vi "Measurement UI.vi"() -> ()   [LabVIEW 2023, in "FPT NoiseFigure UI.lvlib"]
uses:
  FPT NoiseFigure UI.lvlib
  <vilib>/Utility/file.llb/Read Delimited Spreadsheet (DBL).vi
panel:
  in  "Measurement Graph":enum32{"DUT NF", "Separated", "Hidden Controls"}(tab)
  out "Combined Graph":T1(graph)
  out "Graph 2":T1(graph)
  out "Graph 1":T1(graph)
  in  "Power sequencing file validity check":bool=TRUE
  in  "ENS SMU Name":string="5842_0"
  out "DUT NF (mean)":dbl format="%.2g"
  in  "Noise Source Loss S2P File Path":string
  in  "Calibration Loss S2P File Path":string
  in  "DUT Output Loss S2P File Path":string
  in  "DUT Input Loss S2P File Path":string
  out "Analyzer NF vs Freq":dbl[][](array[numeric]) format="%.2g"
  out "DUT NF vs Freq":dbl[][](array[numeric]) format="%.2g"
  in  "Power sequencing file path":string
  in  "RFmx name":string="5842_0"
  in  "RFmx attenuation mode":T2(ring)=enum."Constant Attenuation"
  in  "RFmx s2p file path":string
  out "All Graph Refs":refnum<vi>[](array[refnum])
  in  "ENR Freq (Hz)":dbl[](array[numeric])=[6500000000.0] caption="ENR Freq" format="%.3p Hz"
  in  "ENR (dB)":dbl[](array[numeric])=[15.0] caption="ENR" format="%.2g dB"
  out "Analyzer NF(s)":string[](array[string])
  out "DUT NF(s)":string[](array[string])
  out "Frequencies":string[](array[string])
  out "DUT NF (Mean)":string[](array[string])
  in  "Noise Source Type":i32(ring)=1 items=["External Noise Source", "RF Signal Generator"]
  in  "Switch Name":string
  out "MeasTable 1":string[][](table)
  out "MeasTable 2":string[][](table)
  in  "Action":u32(ring) items=["Measure", "Calibrate"]
  in  "Mode of operation":T3(ring) caption="Configuration"
  in  "Tab Control":T4(tab)
  in  "Power sequencing file path_update":path caption="Power Sequencing File Path"
  in  "RFmx port":string(combo)="port2" caption="RFmx Port"
  in  "RFmx attenuation mode_tab":T2(tab)=enum."s2p File" caption="RFmx Attenuation Mode"
  in  "RFmx external attenuation (dB)":dbl=0.8 caption="External Attenuation" format="%#fdB"
  in  "RFmx s2p file path_update":path caption="S2P File Path"
  in  "RFmx s-parameters orientation":enum32{"Port1 Towards DUT", "Port2 Towards DUT"}(ring) caption="Orientation"
  in  "RFmx name_update":refnum<k15> caption="RFmx Name"
  in  "DUT Output_Orientation":enum32{"Port1 Towards DUT", "Port2 Towards DUT"}(ring) caption="Orientation"
  in  "DUT Input_Orientation":enum32{"Port1 Towards DUT", "Port2 Towards DUT"}(ring) caption="Orientation"
  in  "DUT Output_Compensation Enabled":bool caption="Enabled"
  in  "DUT Input_Compensation Enabled":bool caption="Enabled"
  in  "DUT Input_Temperation (K)":dbl=297.0 caption="Temperature" format="%#fK"
  in  "DUT Output_Temperation (K)":dbl=297.0 caption="Temperature" format="%#fK"
  in  "DUT Input_Loss S2P":path=path "C:/Users/ies-pg-8881/Desktop/KB/CMT/PS_ATT6dB_26.5GHz.csv" caption="DUT Input Loss S2P"
  in  "DUT Output_Loss S2P":path=path "C:/Users/ies-pg-8881/Desktop/KB/CMT/PS_ATT6dB_26.5GHz.csv" caption="DUT Output Loss S2P"
  in  "Noise Source_Orientation":enum32{"Port1 Towards DUT", "Port2 Towards DUT"}(ring) caption="Orientation"
  in  "Calibration_Orientation":enum32{"Port1 Towards DUT", "Port2 Towards DUT"}(ring) caption="Orientation"
  in  "Noise Source_Compensation Enabled":bool caption="Enabled"
  in  "Calibration_Temperation (K)":dbl=297.0 caption="Temperature" format="%#fK"
  in  "Noise Source_Temperation (K)":dbl=297.0 caption="Temperature" format="%#fK"
  in  "Calibration_Compensation Enabled":bool caption="Enabled"
  in  "Calibration_Loss S2P":path=path "C:/Users/ies-pg-8881/Desktop/KB/CMT/PS_ATT6dB_26.5GHz.csv" caption="Calibration Loss S2P"
  in  "Noise Source_Loss S2P":path=path "C:/Users/ies-pg-8881/Desktop/KB/CMT/PS_ATT6dB_26.5GHz.csv" caption="Noise Source Loss S2P"
  in  "Noise Source Type_Tab":T5(tab)=enum."RF Signal Generator" caption="Noise Source Type"
  in  "ENS SMU Channel":string
  in  "ENS SMU name_update":refnum<k15> caption="ENS SMU Name"
  in  "Switch Connection":string
  in  "Switch Name_update":refnum<k15> caption="Switch Name"
  in  "Noise Source RFSG Port":string(combo)="port1" caption="RFSG Port"
  in  "ENR_File Path":path caption="ENR File Path"
  in  "ENR_Values":cluster{"Frequency":dbl, "Value":dbl}[](array[cluster])=[{"Frequency"=6500000000.0, "Value"=15.0}] {"Value" format="%#fdB"; "Frequency" format="%#pHz"}
  in  "Noise Source Off Temperature (K)":dbl=297.0 caption="Off Temp" format="%#fK"
  in  "Noise Source Cold Temperature (K)":dbl=302.8 caption="Cold Temp" format="%#fK"
  in  "Averaging Enabled":bool
  in  "NF Cal Setup ID":string="SNS_PS_6dB_ENR15_26.5GHz_VI" caption="Calibration Setup ID"
  in  "Preamp Enabled":i32(ring)=3 caption="Preamp" items=["Disabled"=0, "Enabled"=1, "Automatic"=3]
  in  "Reference Level (dBm)":dbl caption="Reference Level" format="%#fdBm"
  in  "Reference Level Mode":enum32{"Manual", "Recommend"}(ring)=enum."Recommend"
  in  "DUT Max Noise Figure (dB)":dbl=3.0 caption="DUT Max Noise Figure" format="%#fdB"
  in  "DUT Max Gain (dB)":dbl=17.5 caption="DUT Max Gain" format="%#fdB"
  in  "Measurement Interval (s)":dbl=0.1 caption="Measurement Interval" format="%#ps"
  in  "Measurement Bandwidth (Hz)":dbl=4000000.0 caption="Measurement BW" format="%#pHz"
  in  "Averaging Count":i32=10
  in  "Frequency List Mode":enum32{"Step", "Points", "Frequency List"}(tab) caption="De-embedding"
  in  "Step - Start Frequency":dbl=4000000000.0 caption="Start Frequency" format="%#pHz"
  in  "Step - Stop Frequency":dbl=20000000000.0 caption="Stop Frequency" format="%#pHz"
  in  "Step - Step Size":dbl=1000000000.0 caption="Step Size" format="%#pHz"
  in  "Points - Number of Points":i32=11 caption="Number of Points"
  in  "Points - Stop Frequency":dbl=20000000000.0 caption="Stop Frequency" format="%#pHz"
  in  "Points - Start Frequency":dbl=4000000000.0 caption="Start Frequency" format="%#pHz"
  in  "FreqList - Frequency List":dbl[](array[numeric]) caption="Frequency List" format="%#pHz"
  out "Status":string
  # "DUT Input Compensation"
  # "DUT Output Compensation"
  # "Calibration Compensation"
  # "Noise Source Compensation"
  # "Noise Source"
  # "ENR Frequency"
  # "ENR"
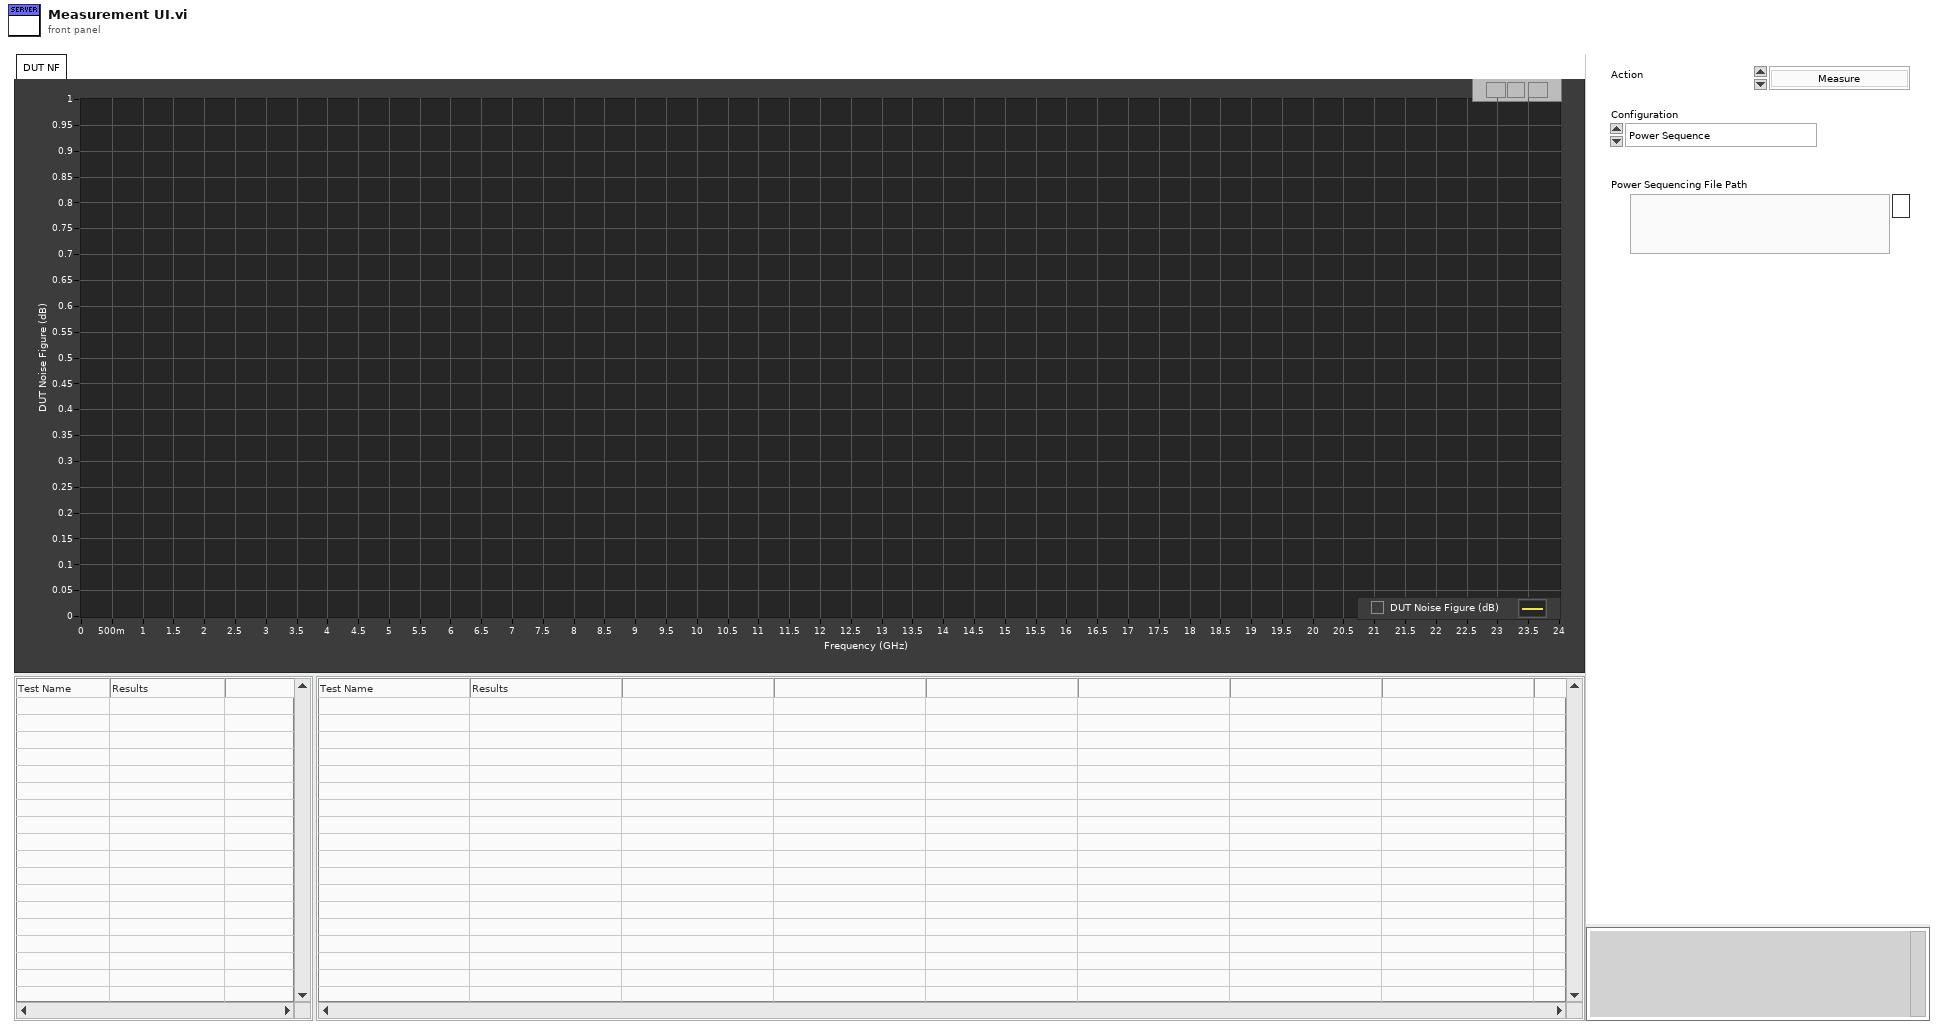
[diagram p1: front panel]
types:
  T1 = cluster{"Load currents":dbl[], "Efficiency":dbl[]}[]
  T2 = enum32{"<None>", "Constant Attenuation", "s2p File"}
  T3 = enum32{"Power Sequence", "HW + De-embedding", "Correction 1", "Correction 2", "Noise Source", "Measurement 1", "Measurement 2"}
  T4 = enum32{"Power Sequence", "De-embedding", "Correction 1", "Correction 2", "Noise Source", "Measurement 1", "Measurement 2"}
  T5 = enum32{"External Noise Source", "RF Signal Generator"}
  T6 = enum16{"<None>", "Constant Attenuation", "s2p File"}
  T7 = enum8{"Enabled", "Disabled", "Disabled and Grayed Out"}
  T8 = cluster{"Shift":bool, "Ctrl":bool, "Alt":bool, "Cmd":bool, "Opt":bool}
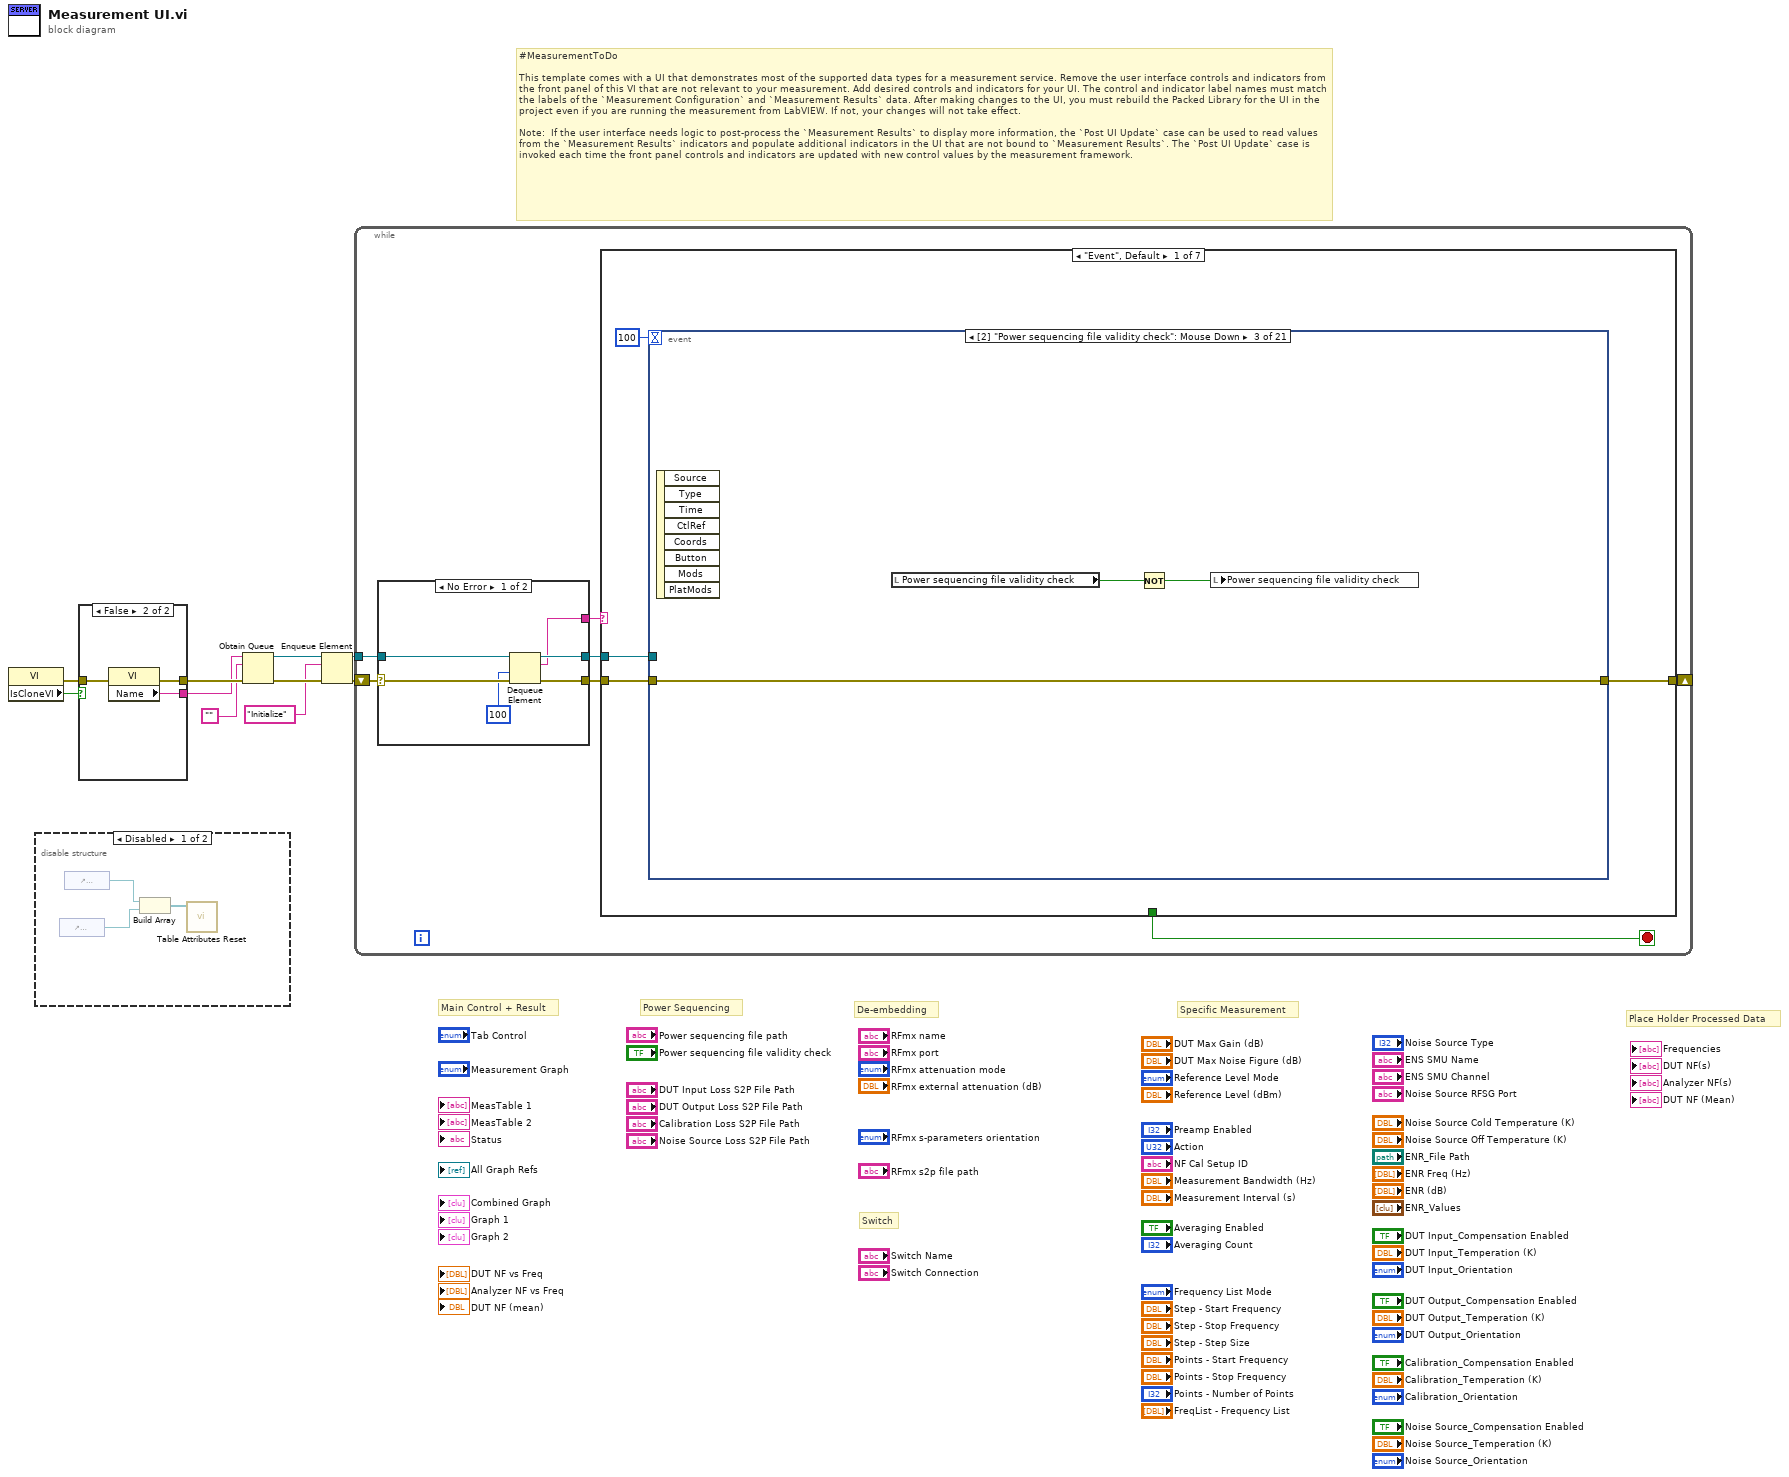
[diagram p0: block diagram]
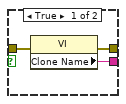
[diagram p3: hidden frame]
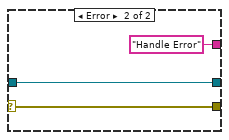
[diagram p4: hidden frame]
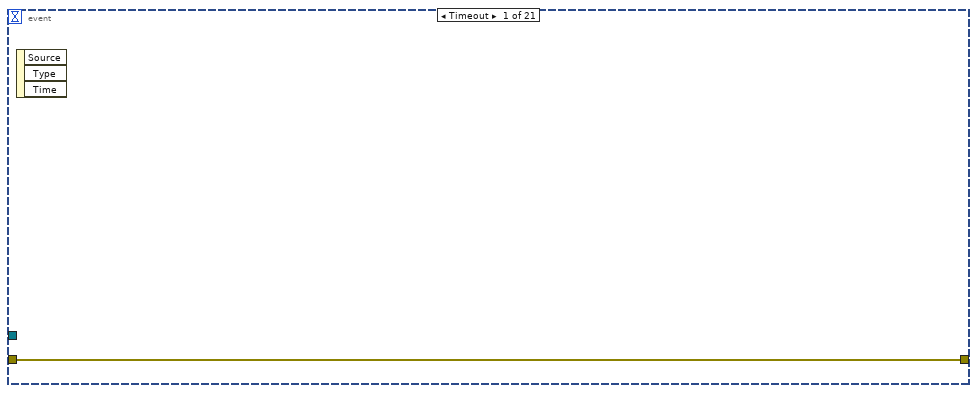
[diagram p5: hidden frame]
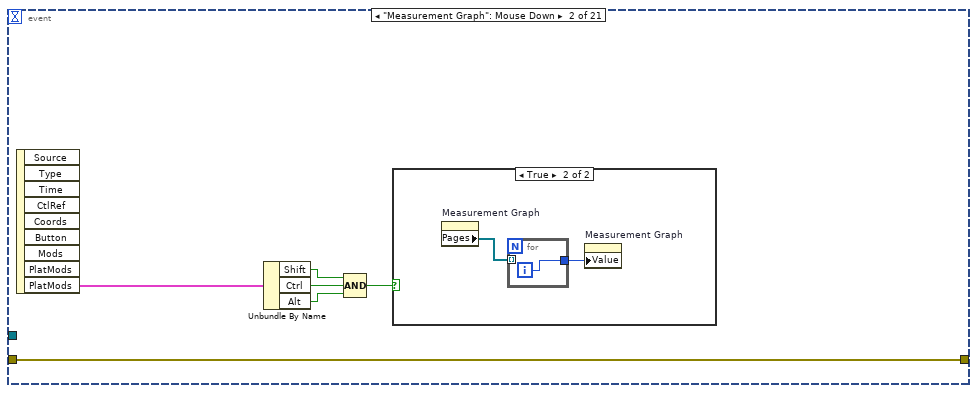
[diagram p6: hidden frame]
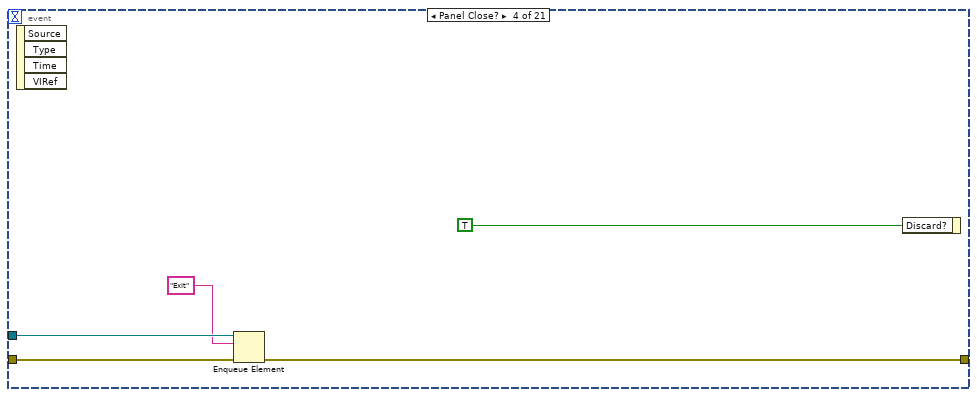
[diagram p8: hidden frame]
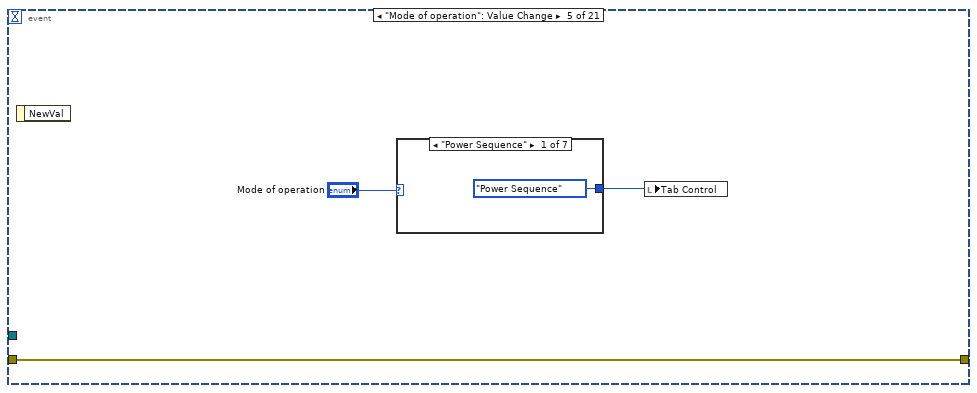
[diagram p9: hidden frame]
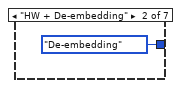
[diagram p10: hidden frame]
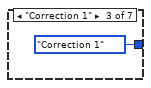
[diagram p11: hidden frame]
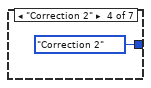
[diagram p12: hidden frame]
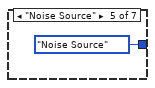
[diagram p13: hidden frame]
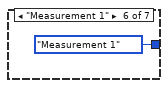
[diagram p14: hidden frame]
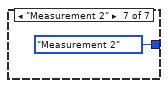
[diagram p15: hidden frame]
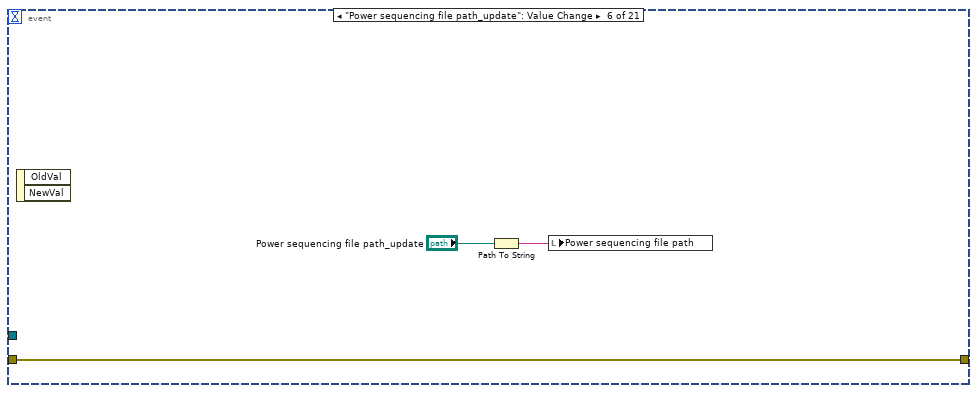
[diagram p16: hidden frame]
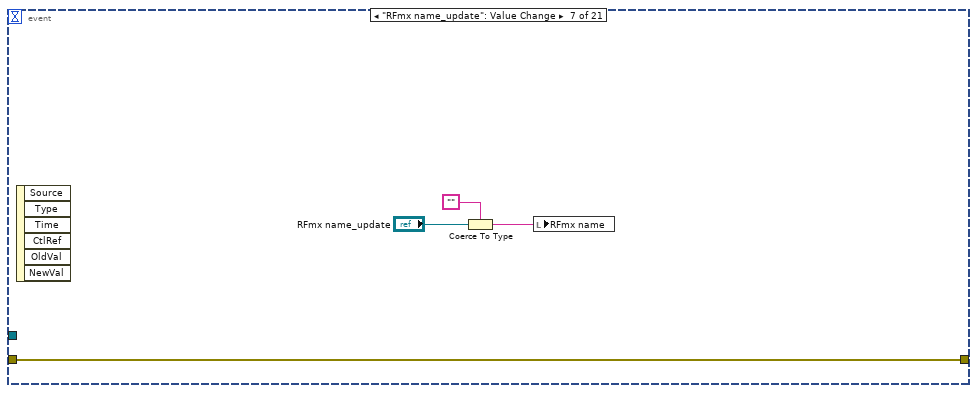
[diagram p17: hidden frame]
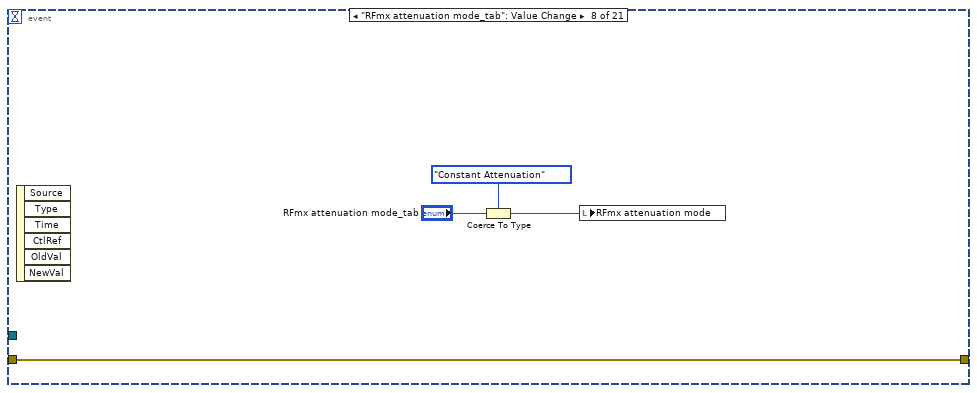
[diagram p18: hidden frame]
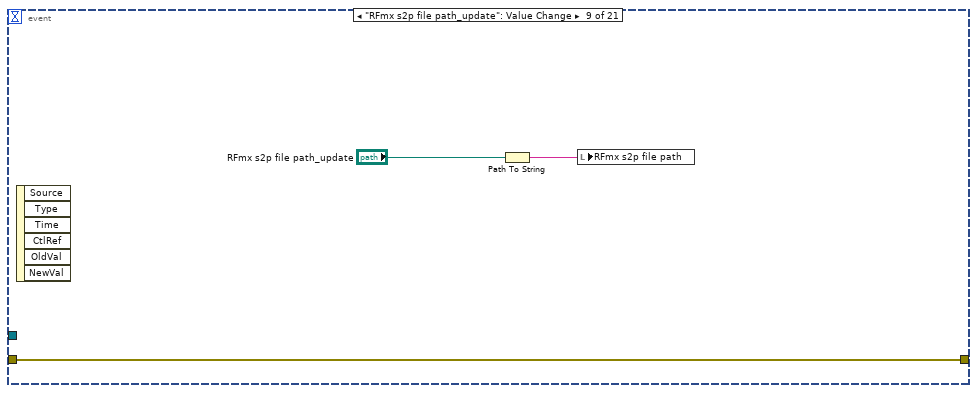
[diagram p19: hidden frame]
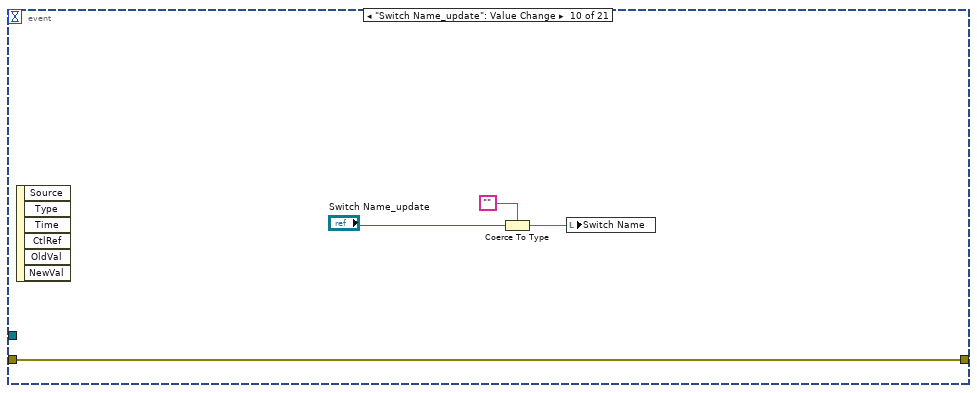
[diagram p20: hidden frame]
diagram:
  # "Switch"
  # "Place Holder Processed Data"
  # "Specific Measurement"
  # "De-embedding"
  # "Power Sequencing"
  # "Main Control + Result"
  # "#MeasurementToDo  \n\nThis template comes with a UI that demonstrates most of the supported data types for a measurement service. Remove the user interface controls and indicators from the front panel of this VI that are not relevant to your measurement. Add desired controls and indicators for your UI. The control and indicator label names must match the labels of the `Measurement Configuration` and `Measurement Results` data. After making changes to the UI, you must rebuild the Packed Library for the UI in the project even if you are running the measurement from LabVIEW. If not, your changes will not take effect.\n\nNote:  If the user interface needs logic to post-process the `Measurement Results` to display more information, the `Post UI Update` case can be used to read values from the `Measurement Results` indicators and populate additional indicators in the UI that are not bound to `Measurement Results`. The `Post UI Update` case is invoked each time the front panel controls and indicators are updated with new control values by the measurement framework."
  n1 = property class="VI"() -> (error out=w1:errorcluster, "IsCloneVI"=w2:bool)  [unwired: 2 in, 1 out]
  n2 = disable-structure shown="Disabled" {
    frame Disabled {
      n3 = control-ref of="MeasTable 2"() -> (w13:refnum<vi>)
      n4 = control-ref of="MeasTable 1"() -> (w12:refnum<vi>)
      n5 = Build Array(w12, w13) -> (w11:refnum<vi>[])
      n6 = call "Table Attributes Reset.vi"("Table Refs"=w11) -> ()  [unwired: 11 in]
    }
    frame Enabled {
    }
  }
  n7 = case shown="False" w2 {
    tunnel: [w16 w19] -> w10
    tunnel: [w15 w18] -> w9
    tunnel: w1 -> [w14 w17]
    frame True {
      n8 = property class="VI"(error in=w14) -> (error out=w16:errorcluster, "Clone Name"=w15:string)  [unwired: 1 in, 1 out]
    }
    frame False {
      n9 = property class="VI"(error in=w17) -> (error out=w19:errorcluster, "Name"=w18:string)  [unwired: 1 in, 1 out]
    }
  }
  n10 = Obtain Queue(name (unnamed)=w9, element data type="", error in (no error)=w10) -> (queue out=w6:refnum<queue>, error out=w8:errorcluster)  [unwired: 2 in, 1 out]
  n11 = Enqueue Element(queue=w6, element="Initialize", error in (no error)=w8) -> (queue out=w5:refnum<queue>, error out=w7:errorcluster)  [unwired: 1 in, 1 out]
  n12 = while {
    shift-right: [w21] -> _
    shift-left: w7 -> [w26]
    tunnel: w5 -> [w24]
    stop <- w20 stop-if-true
    n13 = case shown="No Error" w26 {
      selector: w26 -> [w32 w35]
      tunnel: [w31 w35] -> w25
      tunnel: w24 -> [w30 w34]
      tunnel: [w29 w34] -> w23
      tunnel: [w28 "Handle Error"] -> w22
      frame No Error {
        n14 = Dequeue Element(queue=w30, timeout in ms (-1)=100, error in (no error)=w32) -> (queue out=w29:refnum<queue>, element=w28:string, error out=w31:errorcluster)  [unwired: 1 out]
      }
      frame Error {
      }
    }
    n15 = case shown="\"Event\", Default" w22 {
      tunnel: w25 -> [w38 w161 w211 w238 w242 w253 w254]
      tunnel: w23 -> [w36 _ w210 w237 _ w251 _]
      tunnel: [w39 w161 w211 w239 w244 w248 w254] -> w21
      tunnel: [_ _ _ _ _ TRUE _] -> w20
      frame "Event", Default {
        n16 = event shown="[2] \"Power sequencing file validity check\": Mouse Down" {
          selector: _ -> [_ _ _ _ _ _ _ _ _ _ _ _ _ _ _ _ _ _ _ _ _]
          dyn-events: _ -> [_ _ _ _ _ _ _ _ _ _ _ _ _ _ _ _ _ _ _ _ _]
          timeout: 100 -> [_ _ _ _ _ _ _ _ _ _ _ _ _ _ _ _ _ _ _ _ _]
          tunnel: [w40 w46 w52 w55 w59 w68 w71 w75 w79 w85 w88 w91 w94 w97 w101 w105 w110 w120 w124 w126 w141] -> w39
          tunnel: w38 -> [w40 w46 w52 w56 w59 w68 w71 w75 w79 w85 w88 w91 w94 w97 w101 w105 w110 w121 w124 w126 w145]
          tunnel: w36 -> [_ _ _ w54 _ _ _ _ _ _ _ _ _ _ _ _ _ _ _ _ _]
          event Timeout {
            n17 = event-data() -> ()  [unwired: 1 in, 3 out]
          }
          event "Measurement Graph": Mouse Down {
            n18 = event-data() -> ("PlatMods"=w45:T8)  [unwired: 1 in, 8 out]
            n19 = Unbundle By Name(w45) -> ("Shift"=w44:bool, "Ctrl"=w43:bool, "Alt"=w42:bool)
            n20 = Compound Arithmetic op=AND(w44, w43, w42) -> (w41:bool)
            n21 = case shown="True" w41 {
              frame False {
              }
              frame True {
                n22 = property on="Measurement Graph" class="TabCtl (strict)"() -> ("Pages"=w48:refnum<vi>[])  [unwired: 2 in, 2 out]
                n23 = for {
                  tunnel: [w49] -> w47
                  tunnel: w48 -> [_] mode=indexing
                  i -> [w49]
                }
                n24 = property on="Measurement Graph" class="TabCtl (strict)"("Value"=w47) -> ()  [unwired: 2 in, 2 out]
              }
            }
          }
          event "Power sequencing file validity check": Mouse Down {
            n25 = event-data() -> ()  [unwired: 1 in, 8 out]
            n26 = local read "Power sequencing file validity check"() -> (w51:bool)
            n27 = Not(x=w51) -> (.not. x?=w50:bool)
            n28 = local write "Power sequencing file validity check"(w50) -> ()
          }
          event Panel Close? {
            n29 = event-data() -> ()  [unwired: 1 in, 4 out]
            n30 = Enqueue Element(queue=w54, element="Exit", error in (no error)=w56) -> (error out=w55:errorcluster)  [unwired: 1 in, 2 out]
            n31 = event-data("Discard?"=TRUE) -> ()  [unwired: 1 in, 1 out]
          }
          event "Mode of operation": Value Change {
            n32 = event-data() -> ()  [unwired: 1 in, 1 out]
            n33 = case shown="\"Power Sequence\"" "Mode of operation" {
              tunnel: [T4."Power Sequence" ("Tab Control") T4."De-embedding" ("Tab Control") T4."Correction 1" ("Tab Control") T4."Correction 2" ("Tab Control") T4."Noise Source" ("Tab Control") T4."Measurement 1" ("Tab Control") T4."Measurement 2" ("Tab Control")] -> w58
              frame "Power Sequence" {
              }
              frame "HW + De-embedding" {
              }
              frame "Correction 1" {
              }
              frame "Correction 2" {
              }
              frame "Noise Source" {
              }
              frame "Measurement 1" {
              }
              frame "Measurement 2" {
              }
            }
            n34 = local write "Tab Control"(w58) -> ()
          }
          event "Power sequencing file path_update": Value Change {
            n35 = event-data() -> ()  [unwired: 1 in, 2 out]
            n36 = Path To String(path="Power sequencing file path_update") -> (string=w69:string)
            n37 = local write "Power sequencing file path"(w69) -> ()
          }
          event "RFmx name_update": Value Change {
            n38 = event-data() -> ()  [unwired: 1 in, 6 out]
            n39 = Coerce To Type(0:"RFmx name_update", 1:"") -> (2:w73:string)
            n40 = local write "RFmx name"(w73) -> ()
          }
          event "RFmx attenuation mode_tab": Value Change {
            n41 = event-data() -> ()  [unwired: 1 in, 6 out]
            n42 = Coerce To Type(0:"RFmx attenuation mode_tab", 1:T6."Constant Attenuation" ("RFmx attenuation mode")) -> (2:w76:T6)
            n43 = local write "RFmx attenuation mode"(w76) -> ()
          }
          event "RFmx s2p file path_update": Value Change {
            n44 = event-data() -> ()  [unwired: 1 in, 6 out]
            n45 = Path To String(path="RFmx s2p file path_update") -> (string=w80:string)
            n46 = local write "RFmx s2p file path"(w80) -> ()
          }
          event "Switch Name_update": Value Change {
            n47 = event-data() -> ()  [unwired: 1 in, 6 out]
            n48 = Coerce To Type(0:"Switch Name_update", 1:"") -> (2:w84:string)
            n49 = local write "Switch Name"(w84) -> ()
          }
          event "DUT Input_Loss S2P": Value Change {
            n50 = event-data() -> ()  [unwired: 1 in, 6 out]
            n51 = Path To String(path="DUT Input_Loss S2P") -> (string=w86:string)
            n52 = local write "DUT Input Loss S2P File Path"(w86) -> ()
          }
          event "DUT Output_Loss S2P": Value Change {
            n53 = event-data() -> ()  [unwired: 1 in, 6 out]
            n54 = Path To String(path="DUT Output_Loss S2P") -> (string=w90:string)
            n55 = local write "DUT Output Loss S2P File Path"(w90) -> ()
          }
          event "Calibration_Loss S2P": Value Change {
            n56 = event-data() -> ()  [unwired: 1 in, 6 out]
            n57 = Path To String(path="Calibration_Loss S2P") -> (string=w93:string)
            n58 = local write "Calibration Loss S2P File Path"(w93) -> ()
          }
          event "Noise Source_Loss S2P": Value Change {
            n59 = event-data() -> ()  [unwired: 1 in, 6 out]
            n60 = Path To String(path="Noise Source_Loss S2P") -> (string=w96:string)
            n61 = local write "Noise Source Loss S2P File Path"(w96) -> ()
          }
          event "Noise Source Type_Tab": Value Change {
            w98 = 1 items=["External Noise Source", "RF Signal Generator"] ("Noise Source Type")
            n62 = event-data() -> ()  [unwired: 1 in, 6 out]
            n63 = Coerce To Type(0:"Noise Source Type_Tab", 1:w98) -> (2:w99:i32)
            n64 = local write "Noise Source Type"(w99) -> ()
          }
          event "ENS SMU name_update": Value Change {
            n65 = event-data() -> ()  [unwired: 1 in, 6 out]
            n66 = Coerce To Type(0:"ENS SMU name_update", 1:"") -> (2:w104:string)
            n67 = local write "ENS SMU Name"(w104) -> ()
          }
          event "ENR_Values": Value Change {
            n68 = event-data() -> ("NewVal"=w109:cluster{"Frequency":dbl, "Value":dbl}[])  [unwired: 1 in, 5 out]
            n69 = for {
              tunnel: w109 -> [w113] mode=indexing
              tunnel: [w112] -> w108 mode=indexing
              tunnel: [w111] -> w107 mode=indexing
              n70 = Unbundle By Name(w113) -> ("Frequency"=w112:dbl, "Value"=w111:dbl)
            }
            n71 = local write "ENR (dB)"(w107) -> ()
            n72 = local write "ENR Freq (Hz)"(w108) -> ()
            n73 = local write "ENR_File Path"(path "") -> ()
          }
          event "ENR_File Path": Value Change {
            # "Update the Frequency and Loss/Gain lists based on the selected CSV file"
            n74 = event-data() -> ("NewVal"=w122:path)  [unwired: 1 in, 5 out]
            n75 = call-poly <vilib>:"Read Delimited Spreadsheet.vi"("file path (dialog if empty)"=w122, "error in (no error)"=w121, "delimiter (\\t)"="," ("delimiter (\\t)")) -> ("all rows"=w118:dbl[][], "error out"=w120:errorcluster)  [unwired: 7 in, 4 out]
            n76 = Transpose 2D Array(2D array=w118) -> (transposed array=w117:dbl[][])
            n77 = Index Array(array=w117) -> (element #1=w116:dbl[], element #2=w115:dbl[])  [unwired: 4 in]
            n78 = local write "ENR Freq (Hz)"(w116) -> ()
            n79 = local write "ENR (dB)"(w115) -> ()
            n80 = call "Frequency and Value Arrays to Cluster Array.vi"("Value"=w115, "Frequency"=w116) -> ("Cluster Array"=w114:cluster{"Frequency":dbl, "Value":dbl}[])  [unwired: 9 in]
            n81 = property on="ENR_Values" class="Arr (strict)"("Value"=w114) -> ()  [unwired: 2 in, 2 out]
          }
          event "ENR Freq (Hz)", "ENR (dB)": Value Change {
            # "Reset \"Path Loss File Path\" after manually editing the table"
            n82 = event-data() -> ()  [unwired: 1 in, 6 out]
            n83 = local write "ENR_File Path"(path "" ("DUT Input Loss File Path")) -> ()
          }
          event "Reference Level Mode": Value Change {
            n84 = event-data() -> ("NewVal"=w125:enum32{"Manual", "Recommend"})  [unwired: 1 in, 5 out]
            n85 = case shown="\"Recommend\", Default" w125 {
              frame "Manual" {
                n86 = property on="Reference Level (dBm)" class="DigNum (strict)"("DisabledEnum"=T7."Enabled" ("Disabled")) -> ()  [unwired: 2 in, 2 out]
              }
              frame "Recommend", Default {
                n87 = property on="Reference Level (dBm)" class="DigNum (strict)"("DisabledEnum"=T7."Disabled and Grayed Out" ("Disabled")) -> ()  [unwired: 2 in, 2 out]
              }
            }
          }
          event "Combined Graph", "Graph 1", "Graph 2": Cursor Move {
            # "Update the cursor of specified table(s) based on the dragging cursor"
            n88 = event-data() -> ("CtlRef"=w139:refnum<vi>, "PointIdx"=w133:i32, "CursLoc"=w144:cluster{"X":dbl, "Y":dbl})  [unwired: 1 in, 6 out]
            n89 = property on="All Graph Refs" class="Arr (strict)"() -> ("Value"=w138:refnum<vi>[])  [unwired: 2 in, 2 out]
            n90 = Unbundle By Name(w144) -> ("X"=w135:dbl)
            n91 = Search 1D Array(1D array=w138, element=w139) -> (index of element=w143:i32)  [unwired: 1 in]
            n92 = Delete From Array(array=w138, index=w143) -> (array with subset deleted=w142:refnum<vi>[])  [unwired: 1 in, 1 out]
            n93 = call "Graph Cursor Update.vi"("Action"=enum16{"Reset", "Update"}."Update" ("Cursor to Update"), "error in"=w145, "New X position"=w135, "Cursor Type"=enum16{"Movable", "Fixed", "All"}."Movable", "Graph Refs in"=w142) -> ("error out"=w136:errorcluster)  [unwired: 5 in, 1 out]
            n94 = control-ref of="MeasTable 2"() -> (w129:refnum<vi>)
            n95 = call "Table Highlight.vi"("Action"=enum16{"Reset", "Highlight 1 Row"}."Highlight 1 Row", "error in"=w136, "Color Box"=u32 16776960, "Row"=w133, "Table Ref in"=w129) -> ("error out"=w130:errorcluster)  [unwired: 5 in, 1 out]
            n96 = call <vilib>:"Clear Errors.vi"("error in (no error)"=w130, "specific error code to clear (0: all)"=1055) -> ("error out"=w141:errorcluster)  [unwired: 4 in, 1 out]
          }
        }
      }
      frame "Initialize" {
        w146 = 0
        # "Update array of cluster based on configuration.ctl default values"
        n97 = control-ref of="MeasTable 2"() -> (w157:refnum<vi>)
        n98 = local write "Measurement Graph"(w146) -> ()
        n99 = local write "Tab Control"(w146) -> ()
        n100 = local write "Mode of operation"(w146) -> ()
        n101 = call "Table Highlight.vi"("Action"=enum16{"Reset", "Highlight 1 Row"}."Reset", "Table Ref in"=w157) -> ()  [unwired: 8 in, 2 out]
        n102 = control-ref of="Combined Graph"() -> (w160:refnum<vi>)
        n103 = control-ref of="Graph 1"() -> (w158:refnum<vi>)
        n104 = control-ref of="Graph 2"() -> (w151:refnum<vi>)
        n105 = local read "ENR Freq (Hz)"() -> (w150:dbl[])
        n106 = local read "ENR (dB)"() -> (w149:dbl[])
        n107 = Build Array(w160, w158, w151) -> (w155:refnum<vi>[])
        n108 = property on="Reference Level Mode" class="Enum (strict)"("Val(Sgnl)"=enum32{"Manual", "Recommend"}."Recommend" ("Value (Signaling)")) -> ()  [unwired: 2 in, 2 out]
        n109 = call "Frequency and Value Arrays to Cluster Array.vi"("Value"=w149, "Frequency"=w150) -> ("Cluster Array"=w148:cluster{"Frequency":dbl, "Value":dbl}[])  [unwired: 9 in]
        n110 = property on="All Graph Refs" class="Arr (strict)"("Value"=w155) -> ()  [unwired: 2 in, 2 out]
        n111 = call "Graph Set Cursor Mode.vi"("Cursor Mode"=enum32{"Free-Drag", "Single-Plot", "Multi-Plot"}."Multi-Plot", "Graph Refs in"=w155) -> ("Graph Refs out"=w154:refnum<vi>[])  [unwired: 8 in, 1 out]
        n112 = local write "ENR_Values"(w148) -> ()
        n113 = call "Graph Cursor Update.vi"("Action"=enum16{"Reset", "Update"}."Reset", "Cursor Type"=enum16{"Movable", "Fixed", "All"}."All", "Graph Refs in"=w154) -> ()  [unwired: 7 in, 2 out]
      }
      frame "Post UI Update" {
        # "---------------------Get Analyzer NF(s)---------------------"
        # "-------------Get DUT NF(s) & DUT NF Mean-------------"
        # "---------------------Get Frequencies & DUT NF (s)---------------------"
        # "This case will be triggered, after framework updates the User interface with result values.\nUsed to update data type def"
        n114 = local read "Noise Source Loss S2P File Path"() -> (w183:string)
        n115 = local read "DUT Output Loss S2P File Path"() -> (w185:string)
        n116 = local read "Calibration Loss S2P File Path"() -> (w184:string)
        n117 = local read "DUT Input Loss S2P File Path"() -> (w186:string)
        n118 = local read "Reference Level Mode"() -> (w168:enum32{"Manual", "Recommend"})
        n119 = local read "Power sequencing file path"() -> (w199:string)
        n120 = local read "RFmx s2p file path"() -> (w207:string)
        n121 = local read "RFmx attenuation mode"() -> (w201:T2)
        n122 = local read "Noise Source Type"() -> (w167:i32)
        n123 = local read "Switch Name"() -> (w162:string)
        n124 = local read "RFmx name"() -> (w203:string)
        n125 = local read "ENS SMU Name"() -> (w175:string)
        n126 = Enqueue Element(queue=w210, element="Post UI Update 2") -> ()  [unwired: 2 in, 3 out]
        n127 = local read "ENR Freq (Hz)"() -> (w172:dbl[])
        n128 = case shown="\"Recommend\"" w168 {
          tunnel: [T7."Enabled" ("Disabled") T7."Disabled and Grayed Out" ("Disabled")] -> w169
          frame "Manual", Default {
            # "Manual Ref"
          }
          frame "Recommend" {
            # "Recommended Ref"
          }
        }
        n129 = local read "ENR (dB)"() -> (w171:dbl[])
        n130 = Coerce To Type(0:w201, 1:T2."Constant Attenuation" ("RFmx attenuation mode_tab")) -> (2:w202:T2)
        n131 = Coerce To Type(0:w167, 1:T5."RF Signal Generator" ("Noise Source Type_Tab")) -> (2:w166:T5)
        n132 = String To Path(string=w199) -> (path=w208:path)
        n133 = Coerce To Type(0:w203, 1:refnum<k15> refnum ("RFSG name_update")) -> (2:w205:refnum<k15>)
        n134 = Coerce To Type(0:w162, 1:refnum<k15> refnum ("RFSG name_update")) -> (2:w163:refnum<k15>)
        n135 = String To Path(string=w207) -> (path=w206:path)
        n136 = String To Path(string=w186) -> (path=w190:path)
        n137 = String To Path(string=w185) -> (path=w189:path)
        n138 = String To Path(string=w184) -> (path=w188:path)
        n139 = String To Path(string=w183) -> (path=w187:path)
        n140 = Coerce To Type(0:w175, 1:refnum<k15> refnum ("RFSG name_update")) -> (2:w174:refnum<k15>)
        n141 = local write "Power sequencing file path_update"(w208) -> ()
        n142 = local write "Switch Name_update"(w163) -> ()
        n143 = local write "RFmx name_update"(w205) -> ()
        n144 = local write "RFmx attenuation mode_tab"(w202) -> ()
        n145 = local write "ENS SMU name_update"(w174) -> ()
        n146 = call "Frequency and Value Arrays to Cluster Array.vi"("Value"=w171, "Frequency"=w172) -> ("Cluster Array"=w170:cluster{"Frequency":dbl, "Value":dbl}[])  [unwired: 9 in]
        n147 = local write "Noise Source Type_Tab"(w166) -> ()
        n148 = local write "RFmx s2p file path_update"(w206) -> ()
        n149 = local write "DUT Input_Loss S2P"(w190) -> ()
        n150 = local write "DUT Output_Loss S2P"(w189) -> ()
        n151 = local write "Calibration_Loss S2P"(w188) -> ()
        n152 = local write "Noise Source_Loss S2P"(w187) -> ()
        n153 = local write "ENR_Values"(w170) -> ()
        n154 = property on="Reference Level Mode" class="Enum (strict)"("Val(Sgnl)"=w168) -> ()  [unwired: 2 in, 2 out]
        n155 = property on="Reference Level (dBm)" class="DigNum (strict)"("DisabledEnum"=w169) -> ()  [unwired: 2 in, 2 out]
        n156 = local read "Analyzer NF vs Freq"() -> (w195:dbl[][])
        n157 = local read "DUT NF vs Freq"() -> (w192:dbl[][])
        n158 = local read "DUT NF vs Freq"() -> (w198:dbl[][])
        n159 = local read "DUT NF (mean)"() -> (w176:dbl)
        n160 = Delete From Array(array=w192, index (row)=0) -> (deleted portion=w193:dbl[])  [unwired: 2 in, 1 out]
        n161 = Delete From Array(array=w198, index (row)=1) -> (deleted portion=w182:dbl[])  [unwired: 2 in, 1 out]
        n162 = Delete From Array(array=w195, index (row)=1) -> (deleted portion=w180:dbl[])  [unwired: 2 in, 1 out]
        n163 = Number To Fractional String(number=w193) -> (F-format string=w179:string[])  [unwired: 3 in]
        n164 = Number To Fractional String(number=w182) -> (F-format string=w191:string[])  [unwired: 3 in]
        n165 = Number To Fractional String(number=w180) -> (F-format string=w181:string[])  [unwired: 3 in]
        n166 = Number To Fractional String(number=w176) -> (F-format string=w178:string)  [unwired: 3 in]
        n167 = Build Array(w178) -> (w177:string[])
        n168 = local write "DUT NF (Mean)"(w177) -> ()
        n169 = local write "Frequencies"(w179) -> ()
        n170 = local write "Analyzer NF(s)"(w181) -> ()
        n171 = local write "DUT NF(s)"(w191) -> ()
      }
      frame "Post UI Update 2" {
        # "---------------------Table 1---------------------\n<Freq><DUT NF><Analyzer NF>"
        # "---------------Graph1---------------\nDUT NF vs Freq"
        # "---------------Graph0---------------\nDUT NF vs Freq"
        # "---------------Graph4---------------\nAnalyzer NF vs Freq"
        # "---------------------Table 2---------------------\n<Freq><DUT NF><Analyzer NF>"
        # "Run after Post UI Update. Can be duplicate is need more processing.\nUtilize this case to convert the result to graph or table"
        n172 = local read "Analyzer NF(s)"() -> (w222:string[])
        n173 = local read "Frequencies"() -> (w230:string[])
        n174 = local read "DUT NF(s)"() -> (w223:string[])
        n175 = Enqueue Element(queue=w237, element="Post UI Update 3", error in (no error)=w238) -> (error out=w239:errorcluster)  [unwired: 1 in, 2 out]
        n176 = control-ref of="MeasTable 2"() -> (w231:refnum<vi>)
        n177 = Build Array(w230, w223, w222) -> (w233:string[][])
        n178 = call "Table Set Header Name and Data (String).vi"("Data"=w233, "Header"=string[] ["Frequency (GHz)", "DUT NF (dB)", "Analyzer NF (dB)"], "Table Ref"=w231) -> ()  [unwired: 9 in]
        n179 = local read "DUT NF (Mean)"() -> (w215:string[])
        n180 = control-ref of="MeasTable 1"() -> (w217:refnum<vi>)
        n181 = local read "DUT NF vs Freq"() -> (w234:dbl[][])
        n182 = control-ref of="Combined Graph"() -> (w236:refnum<vi>)
        n183 = Build Array(string[] ["Average"] ("Header"), w215) -> (w216:string[][])
        n184 = call "Table Set Header Name and Data (String).vi"("Data"=w216, "Header"=string[] ["", "DUT NF (dB)"], "Table Ref"=w217) -> ()  [unwired: 9 in]
        n185 = call "Graph Assign Plot Names and Data.vi"("Legend Number of Rows"=1, "X Ys Data"=w234, "Plot Names"=string[] ["DUT Noise Figure (dB)"], "Graph Ref in"=w236) -> ()  [unwired: 5 in, 3 out]
        n186 = local read "Analyzer NF vs Freq"() -> (w224:dbl[][])
        n187 = local read "DUT NF vs Freq"() -> (w229:dbl[][])
        n188 = control-ref of="Graph 1"() -> (w227:refnum<vi>)
        n189 = control-ref of="Graph 2"() -> (w226:refnum<vi>)
        n190 = call "Graph Assign Plot Names and Data.vi"("Legend Number of Rows"=1, "X Ys Data"=w229, "Plot Names"=string[] ["DUT Noise Figure (dB)"], "Graph Ref in"=w227) -> ()  [unwired: 5 in, 3 out]
        n191 = call "Graph Assign Plot Names and Data.vi"("Legend Number of Rows"=1, "X Ys Data"=w224, "Plot Names"=string[] ["Analyzer Noise Figure (dB)"], "Graph Ref in"=w226) -> ()  [unwired: 5 in, 3 out]
      }
      frame "Post UI Update 3" {
        # "Run after Post UI Update. Can be duplicate is need more processing.\nUtilize this case to convert the result to graph or table"
        n192 = property on="All Graph Refs" class="Arr (strict)"() -> ("Value"=w243:refnum<vi>[])  [unwired: 2 in, 2 out]
        n193 = call "Graph Cursor Update.vi"("Action"=enum16{"Reset", "Update"}."Update" ("Cursor to Update"), "error in"=w242, "New X position"=0.0, "Cursor Type"=enum16{"Movable", "Fixed", "All"}."Movable", "Graph Refs in"=w243) -> ("error out"=w244:errorcluster)  [unwired: 5 in, 1 out]
      }
      frame "Exit" {
        # "This case is triggered to close the User Interface from framework"
        n194 = Flush Queue(queue=w251, error in (no error)=w253) -> (queue out=w250:refnum<queue>, error out=w249:errorcluster)  [unwired: 1 out]
        n195 = Release Queue(queue=w250, force destroy? (F)=TRUE, error in (no error)=w249) -> (error out=w248:errorcluster)  [unwired: 2 out]
      }
      frame "Handle Error" {
      }
    }
  }
